vi "ball_tracker.vi"() -> ()   [LabVIEW 2014]
uses:
  <vilib>/event_ctls.llb/eventvkey.ctl
  <vilib>/Utility/inputDevices.llb/mouseAcquire.vi
panel:
  out "Total Movement of Ball, X-Direction":dbl
  out "Total Movement of Ball, Y-Direction":dbl
  # "Hello!\nOnce this program starts (by pressing the white arrow button in the top-left corner), it will take over the mouse.\nDon't panic! \nTo terminate the program, press the Enter or Return key on the keyboard.\nTo reset the counters below, press the Shift key."
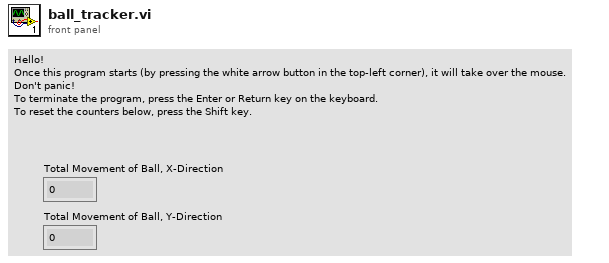
[diagram p1: front panel]
types:
  T1 = typedef "eventvkey.ctl" = enum16{"ASCII", "Enter", "Return", "Shift", "Ctrl", "Alt", "Cmd", "Opt", "Caps", "NumLock", "Clear", "Break", "Up", "Down", "Left", "Right", "Insert", "Delete", "Home", "End", "PageUp", "PageDown", "Escape", "Help", "Pause", "ScrollLock", "F1", "F2", "F3", "F4", "F5", "F6", "F7", "F8", "F9", "F10", "F11", "F12", "F13", "F14", "F15", "F16", "F17", "F18", "F19", "F20", "F21", "F22", "F23", "F24", "Play", "VolumeUp", "VolumeDown", "Mute", "Two Byte Char"}
  T2 = cluster{"Horizontal":i32, "Vertical":i32, "Scrolling":i32}
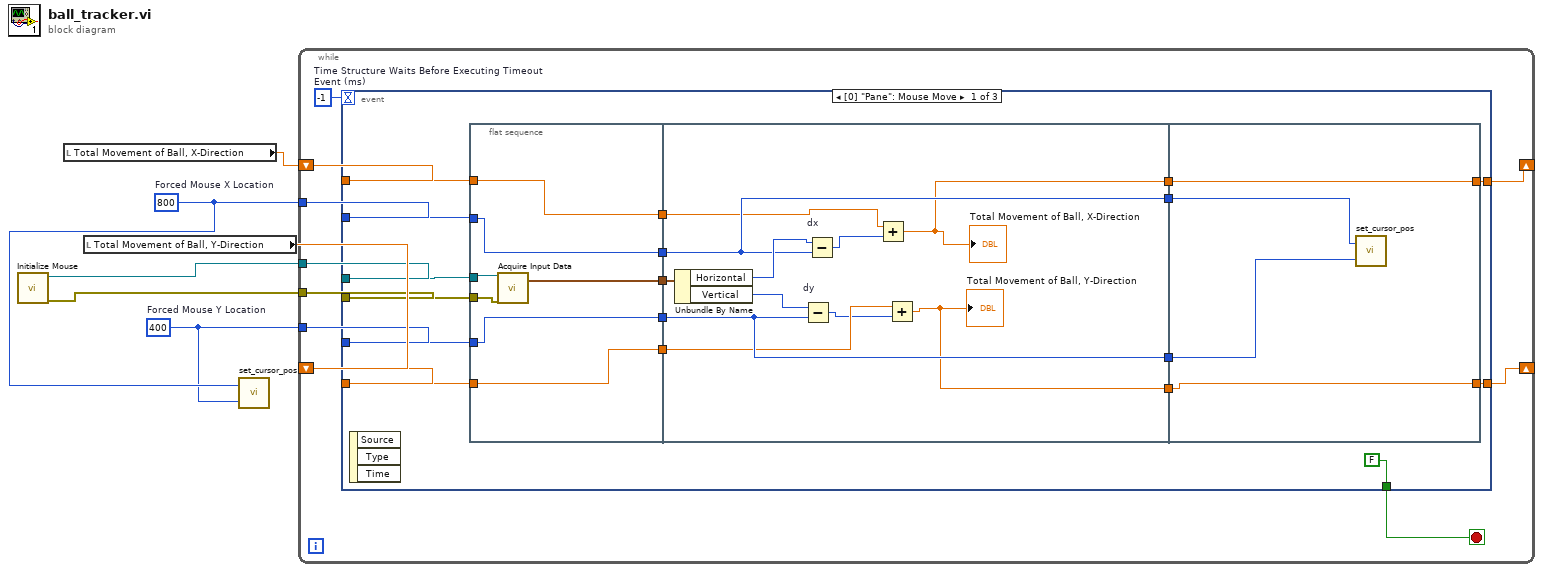
[diagram p0: block diagram]
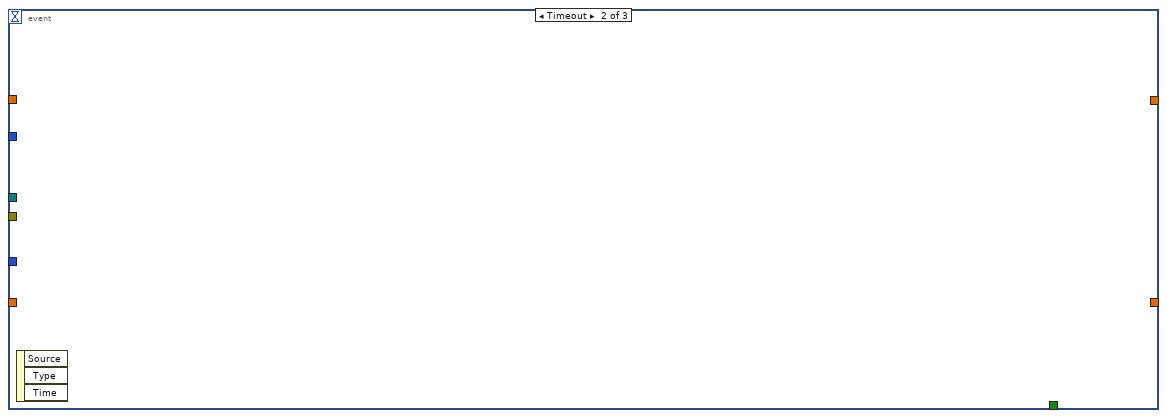
[diagram p2: hidden frame]
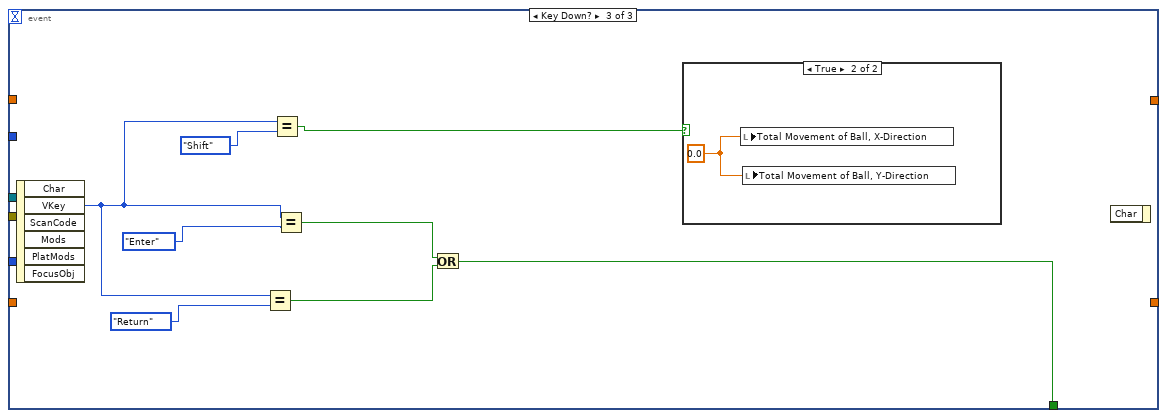
[diagram p3: hidden frame]
diagram:
  w1 = 400  # Forced Mouse Y Location
  w2 = 800  # Forced Mouse X Location
  n1 = call <vilib>:"Initialize Mouse.vi"() -> ("error out"=w6:errorcluster, "device ID"=w5:refnum<k1>)  [unwired: 10 in]
  n2 = local read "Total Movement of Ball, X-Direction"() -> (w4:dbl)
  n3 = local read "Total Movement of Ball, Y-Direction"() -> (w3:dbl)
  n4 = call "set_cursor_pos.vi"("y position"=w1, "x position"=w2) -> ()  [unwired: 1 in]
  n5 = while {
    tunnel: w6 -> [w16]
    tunnel: w5 -> [w15]
    tunnel: w1 -> [w14]
    tunnel: w2 -> [w13]
    shift-right: [w11] -> _
    shift-left: w4 -> [w12]
    shift-right: [w9] -> _
    shift-left: w3 -> [w10]
    stop <- w7 stop-if-true
    w8 = -1  # Time Structure Waits Before Executing Timeout Event (ms)
    n6 = event shown="[0] \"Pane\": Mouse Move" {
      selector: _ -> [_ _ _]
      dyn-events: _ -> [_ _ _]
      timeout: w8 -> [_ _ _]
      tunnel: w16 -> [w25 _ _]
      tunnel: w15 -> [w24 _ _]
      tunnel: w14 -> [w23 _ _]
      tunnel: w13 -> [w22 _ _]
      tunnel: w12 -> [w21 _ _]
      tunnel: [w20 _ _] -> w11
      tunnel: w10 -> [w19 _ _]
      tunnel: [w18 _ _] -> w9
      tunnel: [FALSE _ w60] -> w7
      event Mouse Move {
        n7 = event-data() -> ()  [unwired: 1 in, 3 out]
        n8 = flat-sequence {
          tunnel: w25 -> [w41]
          tunnel: [w40] -> w34
          tunnel: w24 -> [w39]
          tunnel: w22 -> [w38]
          tunnel: [w38] -> w33
          tunnel: w23 -> [w37]
          tunnel: [w37] -> w32
          tunnel: [w36] -> w31
          tunnel: w21 -> [w36]
          tunnel: [w35] -> w30
          tunnel: w19 -> [w35]
          tunnel: w34 -> [w52]
          tunnel: w33 -> [w49]
          tunnel: [w49] -> w29
          tunnel: w32 -> [w48]
          tunnel: [w48] -> w28
          tunnel: w31 -> [w46]
          tunnel: [w45] -> w27
          tunnel: w30 -> [w44]
          tunnel: [w42] -> w26
          tunnel: w29 -> [w56]
          tunnel: w28 -> [w55]
          tunnel: w27 -> [w54]
          tunnel: [w54] -> w20
          tunnel: w26 -> [w53]
          tunnel: [w53] -> w18
          frame #0 {
            n9 = call-poly <vilib>:"Acquire Input Data.vi"("device ID"=w39, "error in (no error)"=w41) -> ("axis info"=w40:T2)  [unwired: 14 in, 3 out]
          }
          frame #1 {
            n10 = Unbundle By Name(w52) -> ("Horizontal"=w51:i32, "Vertical"=w50:i32)
            n11 = Subtract "dy"(x=w50, y=w48) -> (x-y=w43:i32)
            n12 = Subtract "dx"(x=w51, y=w49) -> (x-y=w47:i32)
            n13 = Add(x=w46, y=w47) -> (x+y=w45:dbl)
            "Total Movement of Ball, X-Direction" <- w45
            n14 = Add(x=w44, y=w43) -> (x+y=w42:dbl)
            "Total Movement of Ball, Y-Direction" <- w42
          }
          frame #2 {
            n15 = call "set_cursor_pos.vi"("y position"=w55, "x position"=w56) -> ()  [unwired: 1 in]
          }
        }
      }
      event Timeout {
        n16 = event-data() -> ()  [unwired: 1 in, 3 out]
      }
      event Key Down? {
        n17 = event-data() -> ("VKey"=w58:T1)  [unwired: 1 in, 5 out]
        n18 = Equal?(x=w58, y=eventvkey."Return" ("VKey")) -> (x = y?=w62:bool)
        n19 = Equal?(x=w58, y=eventvkey."Shift" ("VKey")) -> (x = y?=w57:bool)
        n20 = Equal?(x=w58, y=eventvkey."Enter" ("VKey")) -> (x = y?=w61:bool)
        n21 = Or(x=w61, y=w62) -> (x .or. y?=w60:bool)
        n22 = case shown="True" w57 {
          frame False {
          }
          frame True {
            w65 = 0.0 ("Total Movement of Ball, X-Direction")
            n23 = local write "Total Movement of Ball, X-Direction"(w65) -> ()
            n24 = local write "Total Movement of Ball, Y-Direction"(w65) -> ()
          }
        }
        n25 = event-data() -> ()  [unwired: 2 in, 1 out]
      }
    }
  }
